vi "SwapInstanceVIUnusedName2 41.vi"(6 "Bindata & descr in":T1, 7 "type":dbl, 8 "error in (no error)":errorcluster, 9 "dims":u8=3 min=1 max=3, 11 "kwarg_name":string="testarg") -> (0 "error out":errorcluster, 1 "Array 3D":dbl[][][](array[numeric]) format="%.2f", 2 "Array 2D":dbl[][](array[numeric]) format="%.2f", 3 "Array 1D":dbl[](array[numeric]) format="%.2f", 4 "Bindata & descr out":T1, 5 "bindata":u8[](array[numeric]))   [LabVIEW 2018]
uses:
  Bindata&description.ctl
  Bindata description.ctl
  f1c83453-ef33-4fe1-b386-67f83703432c.vi
  8a46b226-3b99-41cc-8c76-34d3a32b2277.vi
  43989767-5720-44c7-93b6-0b6a2919d7cf.vi
  9fed65f7-bb03-4c69-9a7f-41e28756e77e.vi
  8a46b226-3b99-41cc-8c76-34d3a32b2277.vi/842278c5-22e2-4c5f-9198-1cb88e2c7913.vi
  43989767-5720-44c7-93b6-0b6a2919d7cf.vi/3fbea689-4e70-446c-941a-28847dd52786.vi
  9fed65f7-bb03-4c69-9a7f-41e28756e77e.vi/d06b43ce-1229-4c8e-ae12-06e360d86b4b.vi
  8a46b226-3b99-41cc-8c76-34d3a32b2277.vi/842278c5-22e2-4c5f-9198-1cb88e2c7913.vi/7c3e2bfc-f57e-4656-b3d7-5471c41a7a80.vi
  43989767-5720-44c7-93b6-0b6a2919d7cf.vi/3fbea689-4e70-446c-941a-28847dd52786.vi/ba37dff2-851a-4f27-b061-35721d4f87d2.vi
  9fed65f7-bb03-4c69-9a7f-41e28756e77e.vi/d06b43ce-1229-4c8e-ae12-06e360d86b4b.vi/81e6b4db-f1ca-4562-b9cd-32ce0e0334a5.vi
  8a46b226-3b99-41cc-8c76-34d3a32b2277.vi/842278c5-22e2-4c5f-9198-1cb88e2c7913.vi/7c3e2bfc-f57e-4656-b3d7-5471c41a7a80.vi/5dbab519-c520-424a-a111-2dba0746d6c9.vi
  43989767-5720-44c7-93b6-0b6a2919d7cf.vi/3fbea689-4e70-446c-941a-28847dd52786.vi/ba37dff2-851a-4f27-b061-35721d4f87d2.vi/1f70fe1b-f6c9-4ec3-89a2-80c2ccc4b870.vi
  9fed65f7-bb03-4c69-9a7f-41e28756e77e.vi/d06b43ce-1229-4c8e-ae12-06e360d86b4b.vi/81e6b4db-f1ca-4562-b9cd-32ce0e0334a5.vi/f5ddac4b-e08c-43f1-8e9c-0831b4c04b92.vi
  check ID validity.vi
  LV-Julia_ZMQ-Roundtrip_lib.lvlib
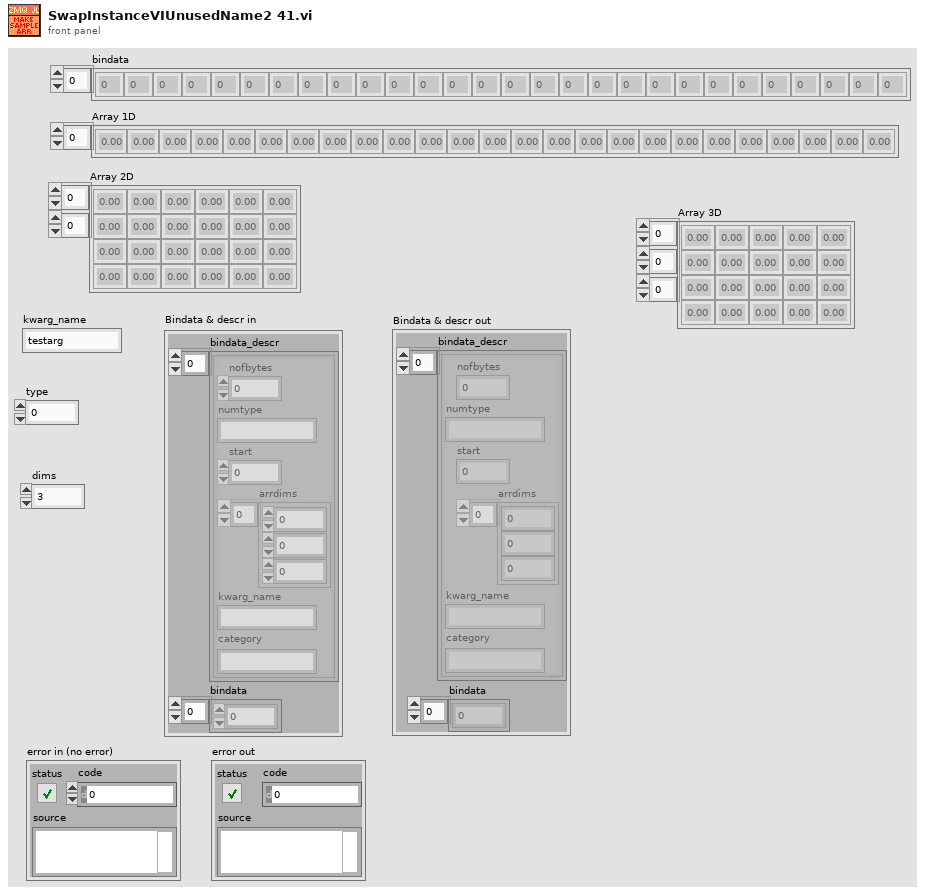
[diagram p1: front panel]
types:
  T1 = typedef "Bindata&description.ctl" = cluster{"bindata_descr":T2[], "bindata":u8[]}
  T2 = typedef "LV-Julia_ZMQ-Roundtrip_lib.lvlib/Bindata description.ctl" = cluster{"nofbytes":i32, "numtype":string, "start":i32, "arrdims":i32[], "kwarg_name":string, "category":string}
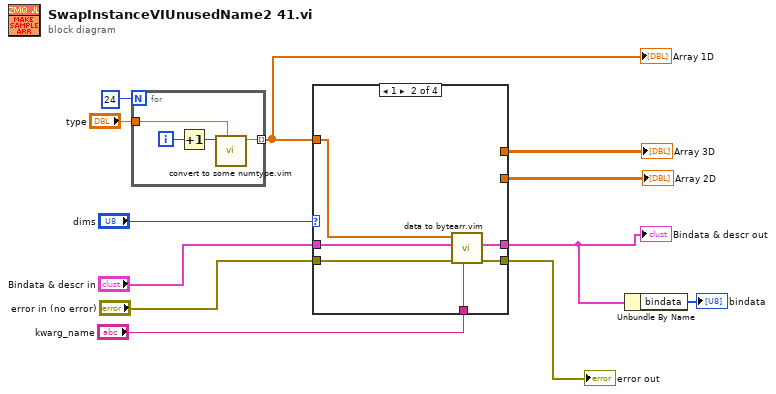
[diagram p0: block diagram]
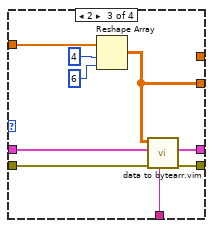
[diagram p3: hidden frame]
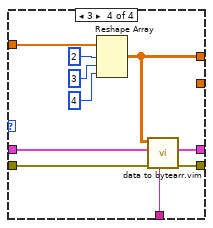
[diagram p4: hidden frame]
diagram:
  n1 = for {
    N: 24 -> [_]
    tunnel: [w14] -> w11 mode=indexing
    tunnel: "type" -> [w13]
    i -> [w16]
    n2 = Increment(x=w16) -> (x+1=w15:i32)
    n3 = call "convert to some numtype.vim"("type"=w13, "Numeric in"=w15) -> ("Numeric out"=w14:dbl)  [unwired: 9 in]
  }
  "Array 1D" <- w11
  n4 = case shown="1" "dims" {
    tunnel: [_ _ _ w42] -> w12
    tunnel: w11 -> [_ w23 w30 w38]
    tunnel: "kwarg_name" -> [_ w22 w29 w37]
    tunnel: "error in (no error)" -> [w17 w21 w28 w36]
    tunnel: [w17 w20 w27 w35] -> w5
    tunnel: [_ w19 w26 w34] -> w2
    tunnel: [_ _ w25 _] -> w4
    tunnel: "Bindata & descr in" -> [_ w18 w24 w33]
    frame 0, Default {
    }
    frame 1 {
      n5 = call "data to bytearr.vim"("kwarg_name"=w22, "error in (no error)"=w21, "Bindata & descr in"=w18, "data in"=w23) -> ("error out"=w20:errorcluster, "Bindata & descr out"=w19:T1)  [unwired: 5 in, 1 out]
    }
    frame 2 {
      n6 = Reshape Array(w30, 4 ("dimension size"), 6 ("dimension size")) -> (w25:dbl[][])
      n7 = call "data to bytearr.vim"("kwarg_name"=w29, "error in (no error)"=w28, "Bindata & descr in"=w24, "data in"=w25) -> ("error out"=w27:errorcluster, "Bindata & descr out"=w26:T1)  [unwired: 5 in, 1 out]
    }
    frame 3 {
      n8 = Reshape Array(w38, 2 ("dimension size"), 3 ("dimension size"), 4 ("dimension size")) -> (w42:dbl[][][])
      n9 = call "data to bytearr.vim"("kwarg_name"=w37, "error in (no error)"=w36, "Bindata & descr in"=w33, "data in"=w42) -> ("error out"=w35:errorcluster, "Bindata & descr out"=w34:T1)  [unwired: 5 in, 1 out]
    }
  }
  "Array 3D" <- w12
  "Bindata & descr out" <- w2
  "error out" <- w5
  "Array 2D" <- w4
  n10 = Unbundle By Name(w2) -> ("bindata"=→"bindata":u8[])
